vi "Untitled 3.vi"() -> ()   [LabVIEW 2020]
uses:
  <vilib>/addons/database/NI_Database_API.lvlib
panel:
  out "columns":string[][](array[string])
  in  "tables 2":string[](array[string])=["OP10_SEALCHECK", "OP20_CONT_TORQ", "OP30_PISTON_ASSY", "OP40_LP", "OP50_HP", "OP60_CSA", "OP70_ASR", "OP80_DRAG", "OP90_DATECODE"]
  out "tables":string[](array[string])
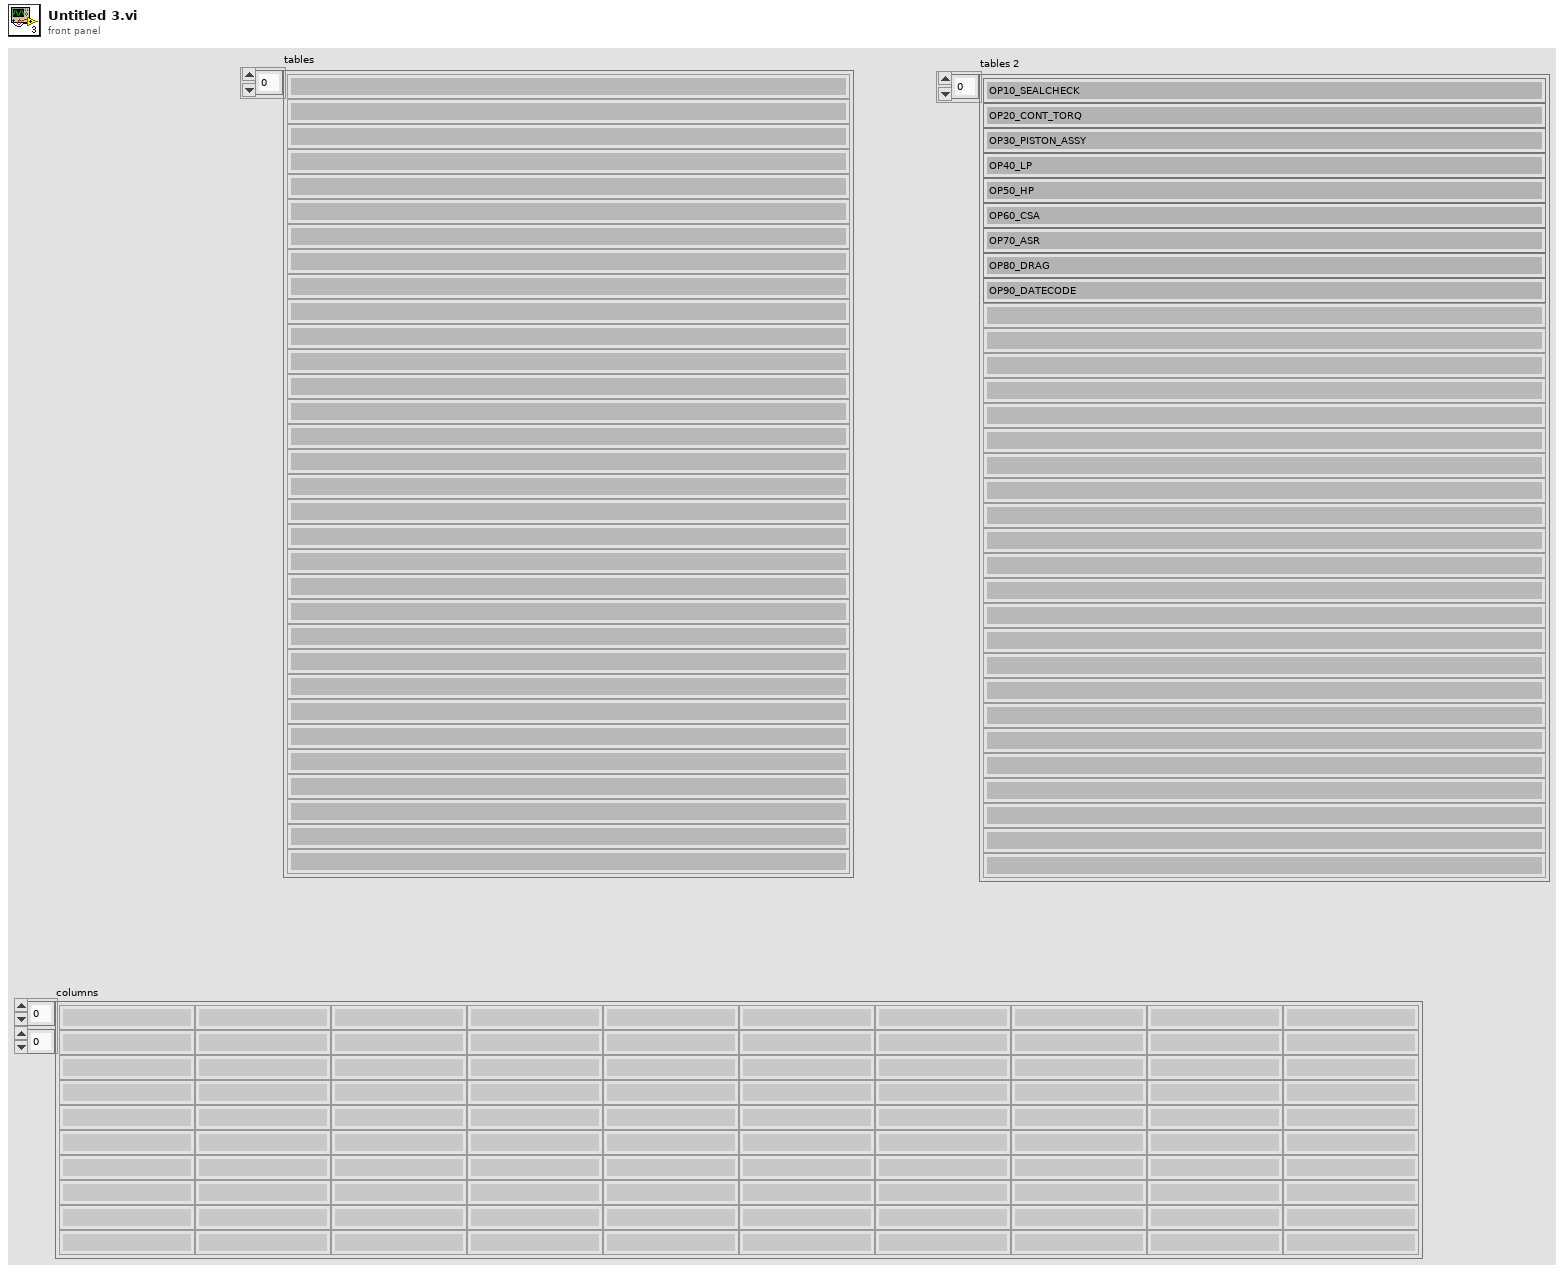
[diagram p1: front panel]
types:
  T1 = typedef "TD SQL.ctl" = cluster{"MS SQL Connection":T2, "UDL File":path, "Time":string, "DCODE":string, "WIP+1":i64, "MC No?":i32, "POKAYOKE?":bool, "Expected Result":string, "Result [Status]":string, "Clock":dbl, "RFID":string, "WIP Queue":refnum<queue>, "TS Parameter":T3, "Data_Queue":refnum<queue>[], "RFID Serial No.":string}
  T2 = typedef "NI_Database_API.lvlib/Conn ObjectReference.ctl" = refnum<k1>
  T3 = typedef "TS_Parameter.ctl" = cluster{"ProfitCenterCode":string, "LineCode":string, "WorkOrderNumber":string, "Model":string, "Model_with_Prefix":string, "VendorCode":string, "SetParameterDateCode":string, "PokaYoke":i32, "Target":i32, "Live_DateCode":string, "CustomerPartNumber":string, "Hand":string, "Ent_Stamp":timestamp, "STS_CD":dbl}
  T4 = cluster{"Data Path":path, "Calibration Path":path, "Settings Path":path, "Script Path":path, "DAQ Support":path, "Reporting Desktop":path, "Help":path}
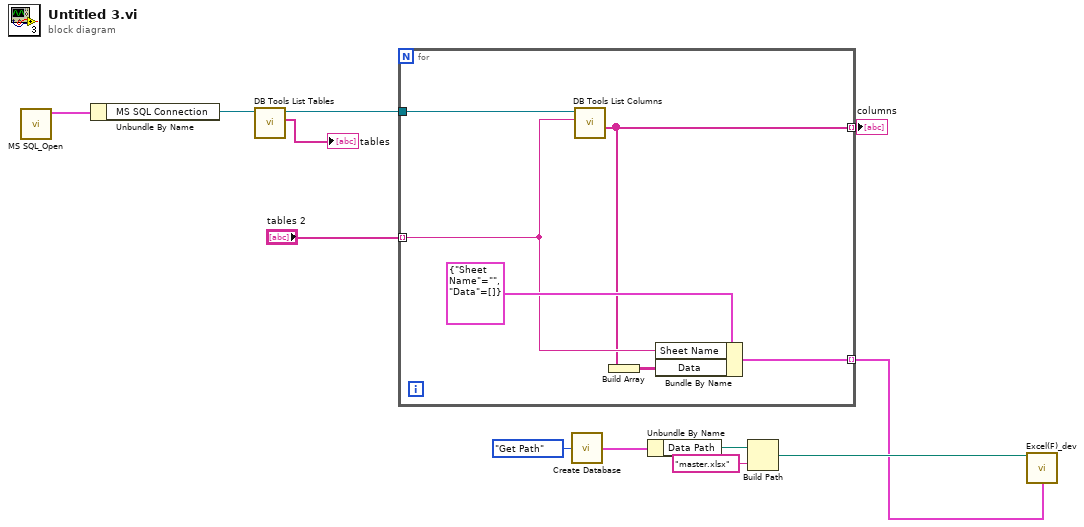
[diagram p0: block diagram]
diagram:
  n1 = call "MS SQL_Open.vi"() -> ("Ref Out"=w12:T1)  [unwired: 9 in, 2 out]
  n2 = Unbundle By Name(w12) -> ("MS SQL Connection"=w11:T2)
  n3 = call <vilib>:"DB Tools List Tables.vi"("connection reference"=w11) -> ("tables"=→"tables":string[], "connection reference out"=w9:T2)  [unwired: 4 in, 1 out]
  n4 = for {
    tunnel: w9 -> [w18]
    tunnel: "tables 2" -> [w16] mode=indexing
    tunnel: [w15] -> w7 mode=indexing
    tunnel: [w13] -> w1 mode=indexing
    n5 = call <vilib>:"DB Tools List Columns.vi"("table"=w16, "connection reference"=w18) -> ("columns"=w15:string[])  [unwired: 2 in, 3 out]
    n6 = Build Array(w15) -> (w14:string[][])
    n7 = Bundle By Name(cluster=cluster{"Sheet Name":string, "Data":string[][]} {"Sheet Name"="", "Data"=[]} ("output cluster"), "Sheet Name"=w16, "Data"=w14) -> (w13:cluster{"Sheet Name":string, "Data":string[][]})
  }
  "columns" <- w7
  n8 = call <userlib>:"Create Database.vi"("Get/Create"=enum16{"Get Path", "Create Path"}."Get Path") -> ("Path Out"=w5:T4)  [unwired: 13 in, 1 out]
  n9 = Unbundle By Name(w5) -> ("Data Path"=w4:path)
  n10 = Build Path(base path=w4, name or relative path="master.xlsx") -> (appended path=w2:path)
  n11 = call "Excel(F)_dev.vi"("Master Path"=w2, "eData"=w1) -> ()  [unwired: 13 in, 1 out]
